vi "Encode UDP Message.vi"(11 "Data":T1={"Command"=enum."Speed", "Msg Length"=0, "Content"=[], "CRC8"=0, "Valid?"=FALSE}) -> (3 "Output string":string)   [LabVIEW 2015]
uses:
  controls/UDP Message Data.ctl
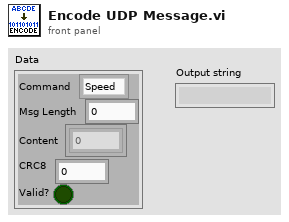
[diagram p1: front panel]
types:
  T1 = typedef "UDP Message Data.ctl" = cluster{"Command":enum16{"Acknowledge", "Speed", "Brake", "Watchdog", "Update", "Unknown", ""}, "Msg Length":u8, "Content":u8[], "CRC8":u8, "Valid?":bool}
  T2 = enum16{"Acknowledge", "Speed", "Brake", "Watchdog", "Update", "Unknown", ""}
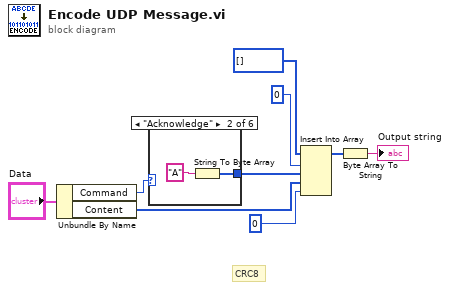
[diagram p0: block diagram]
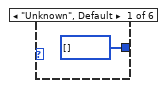
[diagram p2: hidden frame]
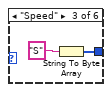
[diagram p3: hidden frame]
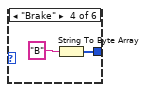
[diagram p4: hidden frame]
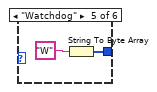
[diagram p5: hidden frame]
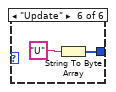
[diagram p6: hidden frame]
diagram:
  # "CRC8"
  n1 = Unbundle By Name("Data") -> ("Command"=w8:T2, "Content"=w5:u8[])
  n2 = case shown="\"Acknowledge\"" w8 {
    tunnel: [u8[] [] ("unsigned byte array") w11 w13 w15 w17 w19] -> w6
    frame "Unknown", Default {
    }
    frame "Acknowledge" {
      n3 = String To Byte Array(string="A") -> (unsigned byte array=w11:u8[])
    }
    frame "Speed" {
      n4 = String To Byte Array(string="S") -> (unsigned byte array=w13:u8[])
    }
    frame "Brake" {
      n5 = String To Byte Array(string="B") -> (unsigned byte array=w15:u8[])
    }
    frame "Watchdog" {
      n6 = String To Byte Array(string="W") -> (unsigned byte array=w17:u8[])
    }
    frame "Update" {
      n7 = String To Byte Array(string="U") -> (unsigned byte array=w19:u8[])
    }
  }
  n8 = Insert Into Array(array=u8[] [], index=0, new element #1=w6, new element #2=w5, new element #3=u8 0 ("new element/subarray")) -> (w2:u8[])
  n9 = Byte Array To String(unsigned byte array=w2) -> (string=→"Output string":string)
